vi "Get Effeciency Test Voltages.vi"(11 "Efficiency Test in":refnum<class "Efficiency Test.lvclass">) -> (3 "Test Voltages":string[](array[string]))   [LabVIEW 2015, in "Efficiency Test.lvclass"]
uses:
  Efficiency Test.lvclass
  Test Class/Test Class.lvclass
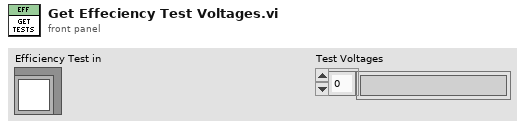
[diagram p1: front panel]
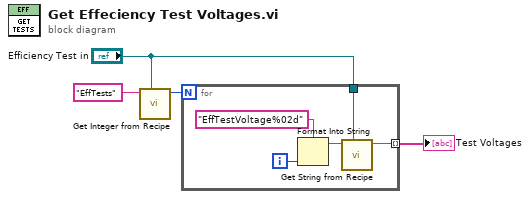
[diagram p0: block diagram]
diagram:
  n1 = call "Get Integer from Recipe.vi"("Test Class in"="Efficiency Test in", "Name"="EffTests") -> ("Value"=w3:i32)  [unwired: 7 in, 2 out]
  n2 = for {
    N: w3 -> [_]
    tunnel: "Efficiency Test in" -> [w9]
    tunnel: [w5] -> w1 mode=indexing
    i -> [w7]
    n3 = Format Into String(format string="EffTestVoltage%02d", w7) -> (resulting string=w6:string)  [unwired: 2 in, 1 out]
    n4 = call "Get String from Recipe.vi"("Test Class in"=w9, "Name"=w6) -> ("Value"=w5:string)  [unwired: 7 in, 2 out]
  }
  "Test Voltages" <- w1
